vi "InputPulseTriggeredOutput_V3_20250127.vi"() -> ()   [LabVIEW 2024]
uses:
  <vilib>/DAQmx/read.llb/DAQmx Read (Analog Wfm 1Chan 1Samp).vi
  <vilib>/DAQmx/write.llb/DAQmx Write (Analog Wfm 1Chan NSamp).vi
  <vilib>/DAQmx/create/channels.llb/DAQmx Create Channel (AI-Voltage-Basic).vi
  <vilib>/DAQmx/configure/timing.llb/DAQmx Timing (Sample Clock).vi
  <vilib>/DAQmx/create/channels.llb/DAQmx Create Channel (AO-Voltage-Basic).vi
  <vilib>/DAQmx/miscellaneous.llb/DAQmx Fill In Error Info.vi
  <vilib>/measure/mamon.llb/Trigger Detection for 1 Channel.vi
  <vilib>/measure/NI_MAPro.lvlib
panel:
  out "data":waveform(dbl)
  in  "stop 2":bool
  in  "stop":bool
  out "trigger detected?":bool
  out "previous stim value":bool
  in  "STIM":bool
  out "Read from DAQ":waveform(dbl)(graph)
  in  "Pulse width 1 (ms)":dbl=1.0 format="%0.2f"
  in  "Amplitude 1":dbl=1.0 format="%0.2p"
  in  "Frequency (Hz)":dbl=1.0 format="%0.2p"
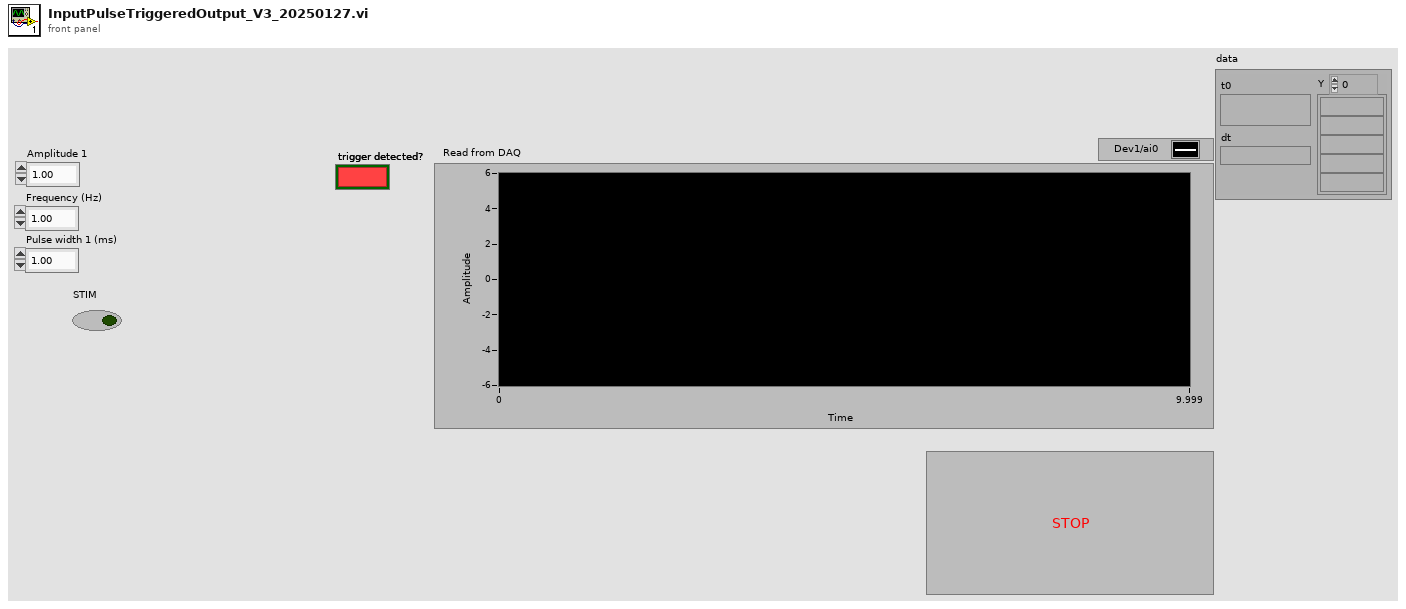
[diagram p1: front panel]
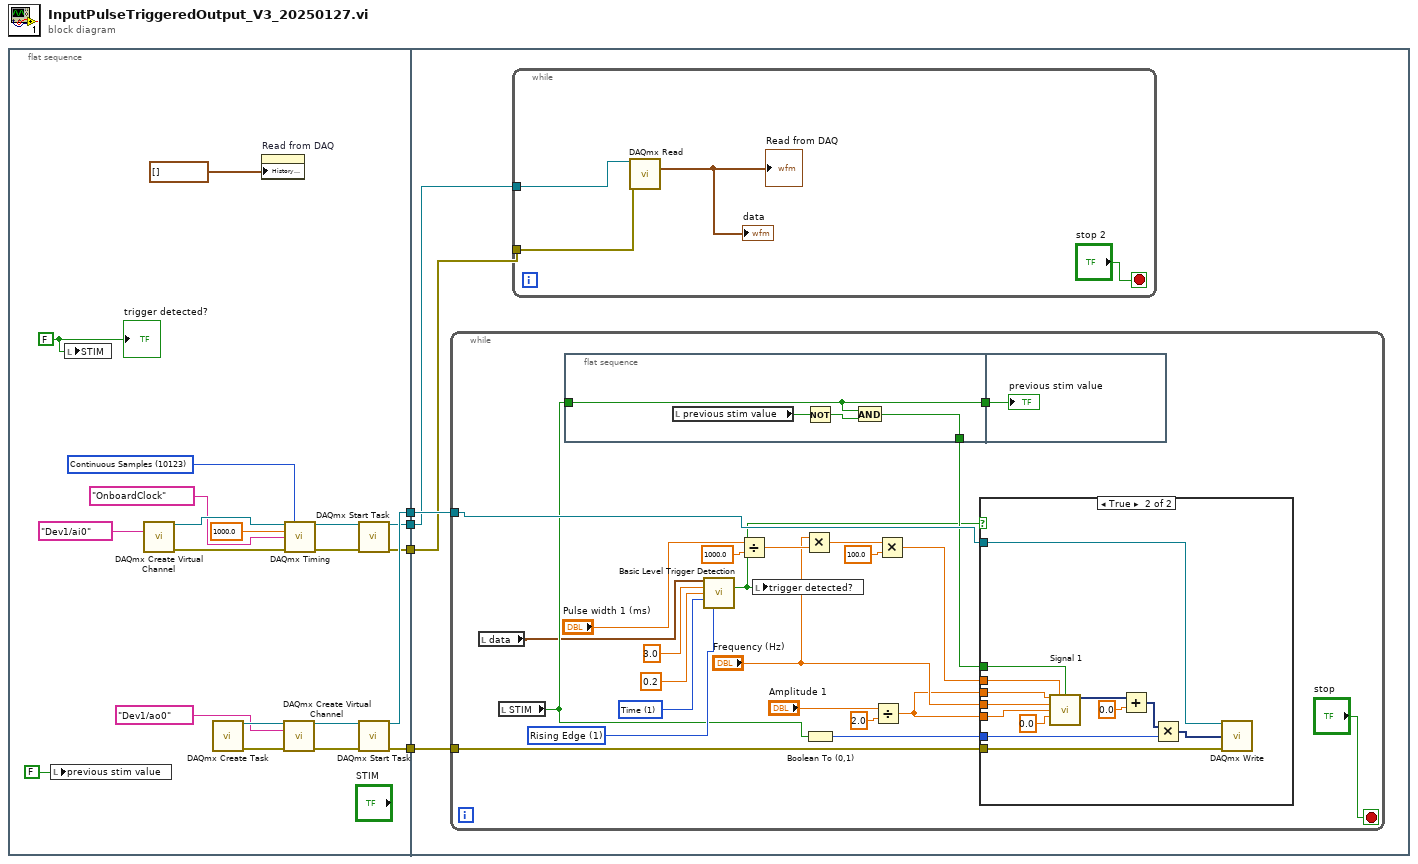
[diagram p0: block diagram]
diagram:
  n1 = flat-sequence {
    tunnel: [w10] -> w4
    tunnel: [w9] -> w3
    tunnel: [w8] -> w2
    tunnel: [w7] -> w1
    tunnel: w4 -> [w28]
    tunnel: w3 -> [w27]
    tunnel: w2 -> [w26]
    tunnel: w1 -> [w25]
    frame #0 {
      w6 = FALSE ("STIM")
      w15 = 10123 items=["Finite Samples"=10178, "Continuous Samples"=10123, "Hardware Timed Single Point"=12522] ("sample mode")
      n2 = local write "previous stim value"(FALSE ("previous stim value")) -> ()
      n3 = local write "STIM"(w6) -> ()
      n4 = call-poly <vilib>:"DAQmx Create Virtual Channel.vi"("physical channels"=tag "Dev1/ai0") -> ("task out"=w16:refnum<k21>, "error out"=w19:errorcluster)  [unwired: 13 in]
      n5 = call <vilib>:"DAQmx Create Task.vi"() -> ("task out"=w21:refnum<k21>, "error out"=w22:errorcluster)  [unwired: 14 in]
      n6 = property on="Read from DAQ" class="WFChart (strict)"("History Data"=waveform(dbl)[] []) -> ()  [unwired: 2 in, 2 out]
      n7 = call-poly <vilib>:"DAQmx Create Virtual Channel.vi"("task in"=w21, "physical channels"=tag "Dev1/ao0", "error in"=w22) -> ("task out"=w23:refnum<k21>, "error out"=w24:errorcluster)  [unwired: 11 in]
      n8 = call-poly <vilib>:"DAQmx Timing.vi"("task/channels in"=w16, "sample mode"=w15, "rate"=1000.0, "source"=tag "OnboardClock", "error in"=w19) -> ("task out"=w17:refnum<k21>, "error out"=w18:errorcluster)  [unwired: 9 in]
      n9 = call <vilib>:"DAQmx Start Task.vi"("task/channels in"=w17, "error in"=w18) -> ("task out"=w8:refnum<k21>, "error out"=w7:errorcluster)  [unwired: 12 in]
      n10 = call <vilib>:"DAQmx Start Task.vi"("task/channels in"=w23, "error in"=w24) -> ("task out"=w10:refnum<k21>, "error out"=w9:errorcluster)  [unwired: 12 in]
      "trigger detected?" <- w6
    }
    frame #1 {
      n11 = while {
        tunnel: w28 -> [w43]
        tunnel: w27 -> [w42]
        stop <- "stop" stop-if-true
        w45 = u16 1 items=["Index", "Time"] ("location mode")
        w44 = u16 1 items=["Falling Edge", "Rising Edge"] ("trigger slope")
        n12 = local read "data"() -> (w33:waveform(dbl))
        n13 = local read "STIM"() -> (w35:bool)
        n14 = flat-sequence {
          tunnel: [w70] -> w55
          tunnel: w35 -> [w70]
          tunnel: [w69] -> w39
          tunnel: w55 -> [w73]
          frame #0 {
            n15 = local read "previous stim value"() -> (w71:bool)
            n16 = Not(x=w71) -> (.not. x?=w72:bool)
            n17 = And(x=w70, y=w72) -> (x .and. y?=w69:bool)
          }
          frame #1 {
            "previous stim value" <- w73
          }
        }
        n18 = call-poly <vilib>:"Basic Level Trigger Detection.vi"("signal in"=w33, "level"=3.0, "hysteresis"=0.2, "location mode"=w45, "trigger slope"=w44) -> ("trigger detected?"=w36:bool)  [unwired: 8 in, 2 out]
        n19 = Divide(x="Pulse width 1 (ms)", y=1000.0) -> (x/y=w50:dbl)
        n20 = local write "trigger detected?"(w36) -> ()
        n21 = Multiply(x="Frequency (Hz)", y=w50) -> (x*y=w48:dbl)
        n22 = Boolean To (0,1)(Boolean=w35) -> (0, 1=w41:i16)
        n23 = Divide(x="Amplitude 1", y=2.0) -> (x/y=w37:dbl)
        n24 = Multiply(x=w48, y=100.0) -> (x*y=w40:dbl)
        n25 = case shown="True" w36 {
          tunnel: w43 -> [_ w65]
          tunnel: w42 -> [_ w64]
          tunnel: w41 -> [_ w62]
          tunnel: w37 -> [_ w61]
          tunnel: w40 -> [_ w60]
          tunnel: w39 -> [_ w59]
          tunnel: "Frequency (Hz)" -> [_ w58]
          tunnel: w37 -> [_ w57]
          frame False {
          }
          frame True {
            n26 = call "Signal 1"("Offset"=w61, "Duty Cycle (%)"=w60, "Reset Signal"=w59, "Frequency"=w58, "Amplitude"=w57, "Phase"=0.0) -> ("Square"=w66:dynamicdata)  [unwired: 8 in, 1 out]
            n27 = Add(x=w66, y=0.0) -> (x+y=w67:dynamicdata)
            n28 = Multiply(x=w67, y=w62) -> (x*y=w68:dynamicdata)
            n29 = call-poly <vilib>:"DAQmx Write.vi"("task/channels in"=w65, "data"=w68, "error in"=w64) -> ()  [unwired: 10 in, 3 out]
          }
        }
      }
      n30 = while {
        tunnel: w26 -> [w30]
        tunnel: w25 -> [w29]
        stop <- "stop 2" stop-if-true
        n31 = call-poly <vilib>:"DAQmx Read.vi"("task/channels in"=w30, "error in"=w29) -> ("data"=→"Read from DAQ" →"data":waveform(dbl))  [unwired: 11 in, 2 out]
      }
    }
  }
